vi "Reposition Legend.vi"(2 "error in (no error)":errorcluster, 3 "Display Type":enum16{"Chart", "Graph"}(ring), 4 "GraphChart in":refnum<vi>) -> (0 "error out":errorcluster, 1 "GraphChart out":refnum<vi>)   [LabVIEW 2015]
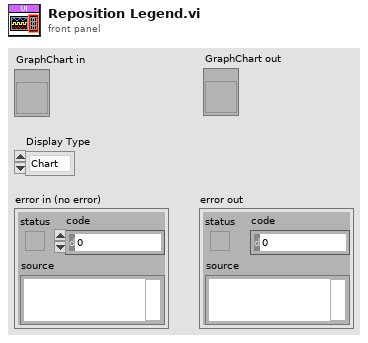
[diagram p1: front panel]
types:
  T1 = typedef "LVBoundsTypeDef.ctl" = cluster{"Width":u32, "Height":u32}
  T2 = typedef "LVPositionTypeDef.ctl" = cluster{"Left":i32, "Top":i32}
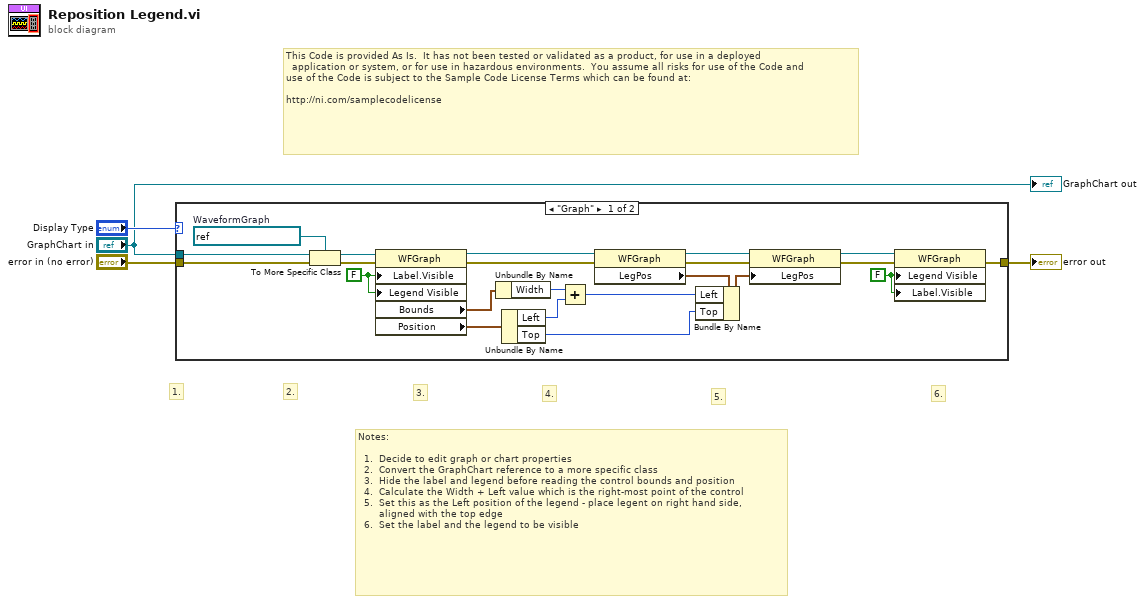
[diagram p0: block diagram]
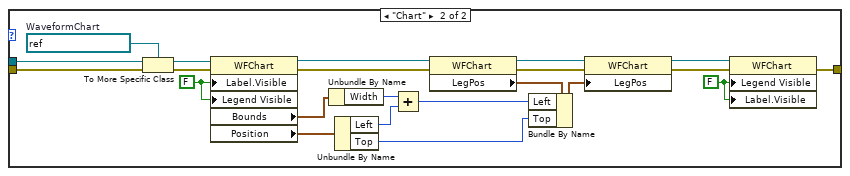
[diagram p2: hidden frame]
diagram:
  # "6."
  # "5."
  # "This Code is provided As Is.  It has not been tested or validated as a product, for use in a deployed\n  application or system, or for use in hazardous environments.  You assume all risks for use of the Code and   \nuse of the Code is subject to the Sample Code License Terms which can be found at: \n\nhttp://ni.com/samplecodelicense"
  # "Notes:  \n\n  1.  Decide to edit graph or chart properties  \n  2.  Convert the GraphChart reference to a more specific class\n  3.  Hide the label and legend before reading the control bounds and position  \n  4.  Calculate the Width + Left value which is the right-most point of the control  \n  5.  Set this as the Left position of the legend - place legent on right hand side,\n       aligned with the top edge\n  6.  Set the label and the legend to be visible"
  # "4."
  # "3."
  # "2."
  # "1."
  n1 = case shown="\"Graph\"" "Display Type" {
    tunnel: [w18 w40] -> w3
    tunnel: "GraphChart in" -> [w7 w29]
    tunnel: "error in (no error)" -> [w6 w28]
    frame "Graph" {
      w5 = FALSE ("Legend:Visible")
      w20 = FALSE ("Legend:Visible")
      w26 = refnum<vi> refnum  # WaveformGraph
      n2 = To More Specific Class(target class=w26, reference=w7, error in=w6) -> (specific class reference=w11:refnum<vi>, error out=w8:errorcluster)
      n3 = property class="WFGraph"(reference=w11, error in=w8, "Label.Visible"=w5, "Legend Visible"=w5) -> (reference out=w10:refnum<vi>, error out=w9:errorcluster, "Bounds"=w17:T1, "Position"=w16:T2)
      n4 = Unbundle By Name(w17) -> ("Width"=w15:u32)
      n5 = Unbundle By Name(w16) -> ("Left"=w14:i32, "Top"=w12:i32)
      n6 = Add(x=w15, y=w14) -> (x+y=w13:u32)
      n7 = property class="WFGraph"(reference=w10, error in=w9) -> (reference out=w24:refnum<vi>, error out=w23:errorcluster, "LegPos"=w22:T2)
      n8 = Bundle By Name(cluster=w22, "Left"=w13, "Top"=w12) -> (w25:T2)
      n9 = property class="WFGraph"(reference=w24, error in=w23, "LegPos"=w25) -> (reference out=w21:refnum<vi>, error out=w19:errorcluster)
      n10 = property class="WFGraph"(reference=w21, error in=w19, "Legend Visible"=w20, "Label.Visible"=w20) -> (error out=w18:errorcluster)  [unwired: 1 out]
    }
    frame "Chart" {
      w27 = FALSE ("Legend:Visible")
      w42 = FALSE ("Legend:Visible")
      w48 = refnum<vi> refnum  # WaveformChart
      n11 = To More Specific Class(target class=w48, reference=w29, error in=w28) -> (specific class reference=w33:refnum<vi>, error out=w30:errorcluster)
      n12 = property class="WFChart"(reference=w33, error in=w30, "Label.Visible"=w27, "Legend Visible"=w27) -> (reference out=w32:refnum<vi>, error out=w31:errorcluster, "Bounds"=w39:T1, "Position"=w38:T2)
      n13 = Unbundle By Name(w39) -> ("Width"=w37:u32)
      n14 = Unbundle By Name(w38) -> ("Left"=w36:i32, "Top"=w34:i32)
      n15 = Add(x=w37, y=w36) -> (x+y=w35:u32)
      n16 = property class="WFChart"(reference=w32, error in=w31) -> (reference out=w46:refnum<vi>, error out=w45:errorcluster, "LegPos"=w44:T2)
      n17 = Bundle By Name(cluster=w44, "Left"=w35, "Top"=w34) -> (w47:T2)
      n18 = property class="WFChart"(reference=w46, error in=w45, "LegPos"=w47) -> (reference out=w43:refnum<vi>, error out=w41:errorcluster)
      n19 = property class="WFChart"(reference=w43, error in=w41, "Legend Visible"=w42, "Label.Visible"=w42) -> (error out=w40:errorcluster)  [unwired: 1 out]
    }
  }
  "error out" <- w3
  "GraphChart out" <- "GraphChart in"
